vi "niRFUtil MT UTIL Generate Filter Coefficients.vi"(0 "System Filter Characteristic (none)":T1(ring), 1 "Modulation Type":T2(ring), 5 "Modulation Samples Per Symbol (16)":i32=16, 7 "Demodulation Samples Per Symbol (16)":i32=16, 9 "Filter Parameter":dbl=0.5 format="%.2f", 11 "error in (no error)":errorcluster, 12 "Filter Length (3)":i32=3) -> (4 "Pulse Shaping Filter Coefficients":T3 min=0 max=127 format="%.2f", 6 "Matched Filter Coefficients":T3 min=0 max=127 format="%.2f", 15 "error out":errorcluster)   [LabVIEW 2015, in "niRFUtil.lvlib"]
uses:
  niRFUtil.lvlib
  Includes/niRFUtil INC Real Array.ctl
  <vilib>/Analysis/2dsp.llb/1D Convolution (DBL).vi
  <vilib>/measure/masml.llb/ma_sml_Interpolation by Zero Insert (real input).vi
  <vilib>/Analysis/NI_AALPro.lvlib
  <vilib>/measure/NI_MAPro.lvlib
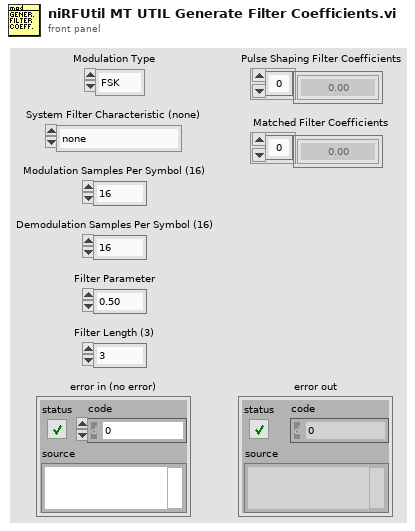
[diagram p1: front panel]
types:
  T1 = enum16{"none", "Raised Cosine", "Root Raised Cos", "Gaussian"}
  T2 = enum16{"FSK", "PSK", "QAM", "MSK", "PAM", "ASK", "CPM"}
  T3 = typedef "niRFUtil.lvlib/niRFUtil INC Real Array.ctl" = sgl[]
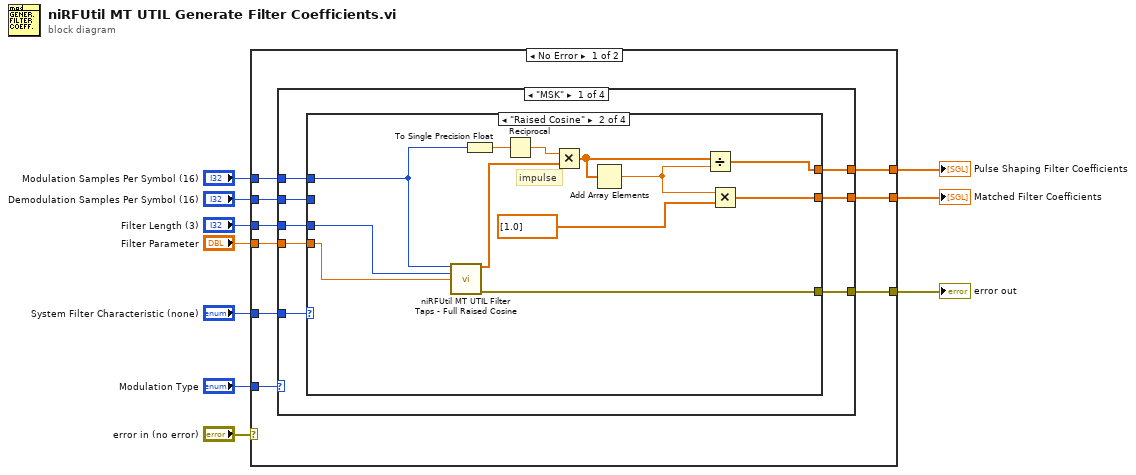
[diagram p0: block diagram]
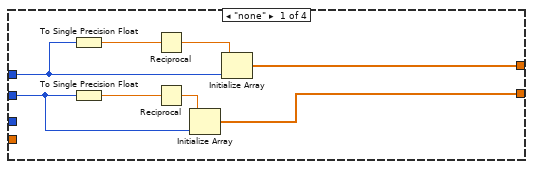
[diagram p2: hidden frame]
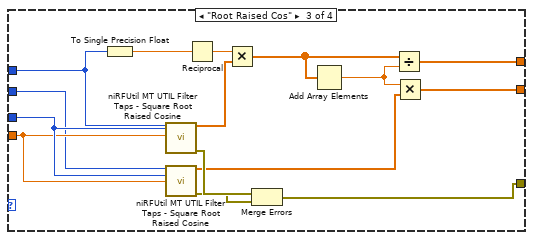
[diagram p3: hidden frame]
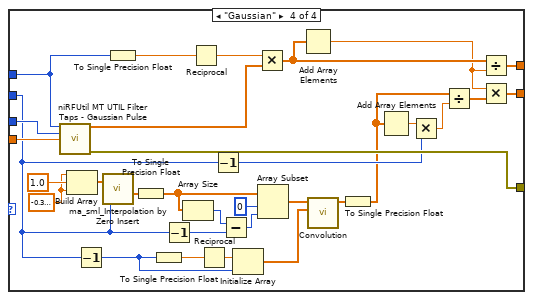
[diagram p4: hidden frame]
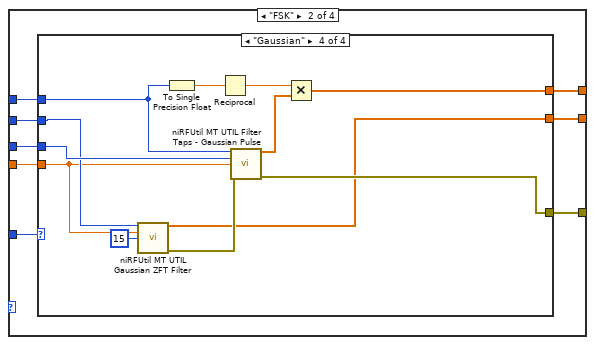
[diagram p5: hidden frame]
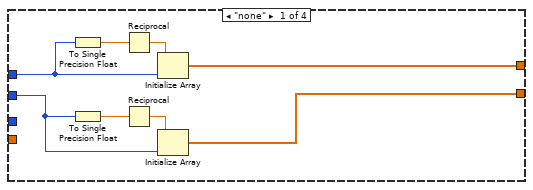
[diagram p6: hidden frame]
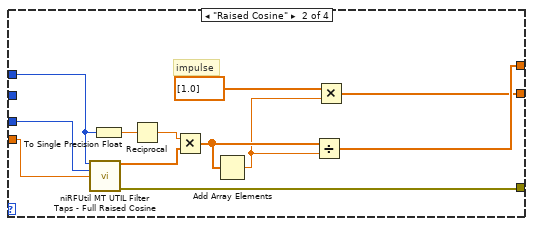
[diagram p7: hidden frame]
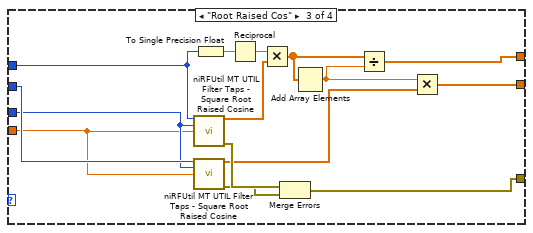
[diagram p8: hidden frame]
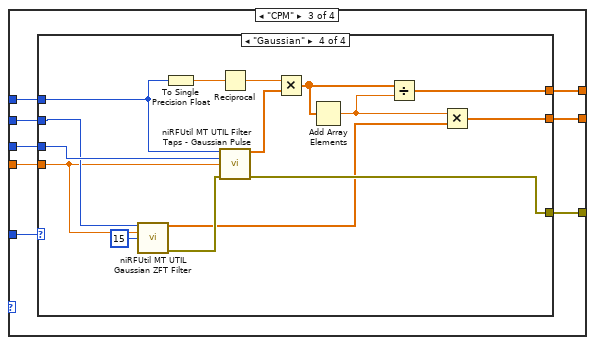
[diagram p9: hidden frame]
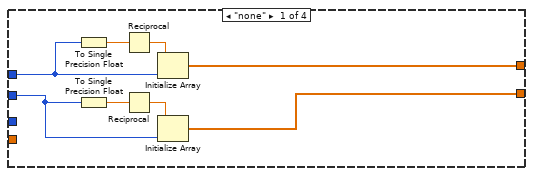
[diagram p10: hidden frame]
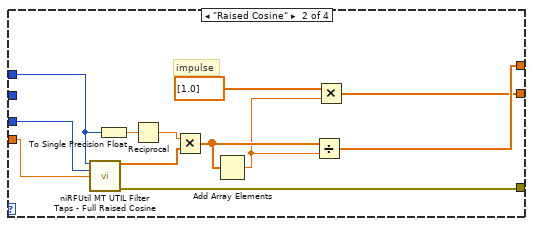
[diagram p11: hidden frame]
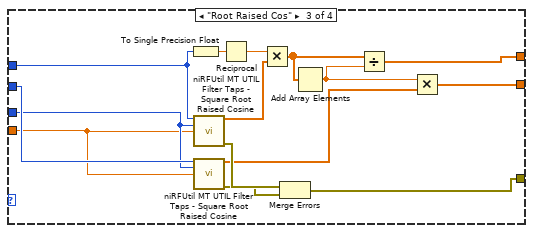
[diagram p12: hidden frame]
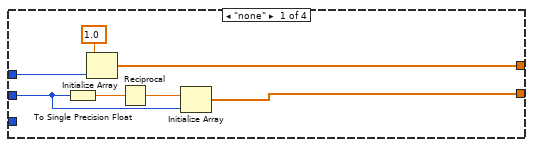
[diagram p14: hidden frame]
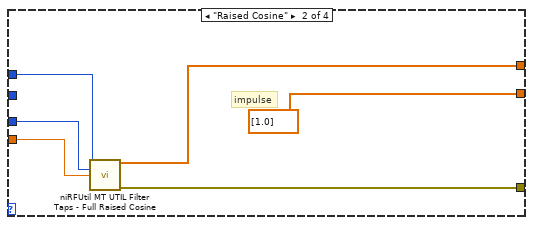
[diagram p15: hidden frame]
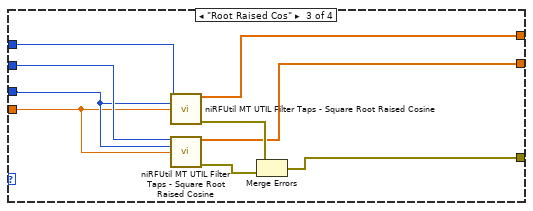
[diagram p16: hidden frame]
diagram:
  n1 = case shown="No Error" "error in (no error)" {
    selector: "error in (no error)" -> [_ w238]
    tunnel: [w19 _] -> w10
    tunnel: [w18 _] -> w9
    tunnel: "Demodulation Samples Per Symbol (16)" -> [w17 _]
    tunnel: "Modulation Type" -> [w16 _]
    tunnel: [w15 w238] -> w6
    tunnel: "Filter Parameter" -> [w14 _]
    tunnel: "Filter Length (3)" -> [w13 _]
    tunnel: "System Filter Characteristic (none)" -> [w12 _]
    tunnel: "Modulation Samples Per Symbol (16)" -> [w11 _]
    frame No Error {
      n2 = case shown="\"MSK\"" w16 {
        tunnel: w11 -> [w27 w102 w157 w215]
        tunnel: w12 -> [w26 w101 w156 w214]
        tunnel: w13 -> [w25 w100 w155 w213]
        tunnel: [w24 w99 w154 w212] -> w18
        tunnel: w14 -> [w23 w98 w153 w211]
        tunnel: [w22 w97 w152 w210] -> w15
        tunnel: w17 -> [w21 w96 w151 w209]
        tunnel: [w20 w95 w150 w208] -> w19
        frame "MSK" {
          n3 = case shown="\"Raised Cosine\"" w26 {
            tunnel: w27 -> [w30 w37 w49 w63]
            tunnel: w25 -> [_ w44 w59 w91]
            tunnel: w23 -> [_ w43 w58 w83]
            tunnel: [_ w45 w57 w93] -> w22
            tunnel: [w35 w41 w54 w71] -> w24
            tunnel: w21 -> [w29 _ w56 w76]
            tunnel: [w34 w38 w51 w70] -> w20
            frame "none" {
              n4 = To Single Precision Float(number=w30) -> (single precision float=w31:sgl)
              n5 = To Single Precision Float(number=w29) -> (single precision float=w28:sgl)
              n6 = Reciprocal(x=w31) -> (1/x=w33:sgl)
              n7 = Reciprocal(x=w28) -> (1/x=w32:sgl)
              n8 = Initialize Array(w32, w29) -> (w34:sgl[])
              n9 = Initialize Array(w33, w30) -> (w35:sgl[])
            }
            frame "Raised Cosine" {
              # "impulse"
              n10 = call "niRFUtil MT UTIL Filter Taps - Full Raised Cosine.vi"("Samples Per Symbol (16)"=w37, "Filter Length (3)"=w44, "Alpha (0.5)"=w43) -> ("Filter Coefficients"=w47:T3, "error out"=w45:errorcluster)  [unwired: 1 in, 10 out]
              n11 = To Single Precision Float(number=w37) -> (single precision float=w36:sgl)
              n12 = Reciprocal(x=w36) -> (1/x=w46:sgl)
              n13 = Multiply(x=w46, y=w47) -> (x*y=w42:T3)
              n14 = Add Array Elements(numeric array=w42) -> (sum=w40:sgl)
              n15 = Divide(x=w42, y=w40) -> (x/y=w41:T3)
              n16 = Multiply(x=w40, y=T3 [1.0]) -> (x*y=w38:T3)
            }
            frame "Root Raised Cos" {
              n17 = To Single Precision Float(number=w49) -> (single precision float=w48:sgl)
              n18 = call "niRFUtil MT UTIL Filter Taps - Square Root Raised Cosine.vi"("Samples Per Symbol (16)"=w49, "Filter Length (3)"=w59, "Alpha (0.5)"=w58) -> ("Filter Coefficients"=w55:T3, "error out"=w62:errorcluster)  [unwired: 1 in, 10 out]
              n19 = call "niRFUtil MT UTIL Filter Taps - Square Root Raised Cosine.vi"("Samples Per Symbol (16)"=w56, "Filter Length (3)"=w59, "Alpha (0.5)"=w58) -> ("Filter Coefficients"=w52:T3, "error out"=w61:errorcluster)  [unwired: 1 in, 10 out]
              n20 = Reciprocal(x=w48) -> (1/x=w60:sgl)
              n21 = Multiply(x=w60, y=w55) -> (x*y=w50:T3)
              n22 = Merge Errors(w62, w61) -> (w57:errorcluster)
              n23 = Add Array Elements(numeric array=w50) -> (sum=w53:sgl)
              n24 = Divide(x=w50, y=w53) -> (x/y=w54:T3)
              n25 = Multiply(x=w53, y=w52) -> (x*y=w51:T3)
            }
            frame "Gaussian" {
              w73 = sgl -0.3
              n26 = call "niRFUtil MT UTIL Filter Taps - Gaussian Pulse.vi"("Samples Per Symbol (16)"=w63, "Filter Length (3)"=w91, "Alpha (0.5)"=w83) -> ("Filter Coefficients"=w94:T3, "error out"=w93:errorcluster)  [unwired: 1 in, 10 out]
              n27 = Build Array(w73, sgl 1.0, w73) -> (w82:sgl[])
              n28 = Decrement(x=w76) -> (x-1=w66:i32)
              n29 = call-poly <vilib>:"ma_sml_Interpolation by Zero Insert.vi"("L"=w76, "x"=w82) -> ("y"=w87:dbl[])
              n30 = To Single Precision Float(number=w63) -> (single precision float=w64:sgl)
              n31 = To Single Precision Float(number=w87) -> (single precision float=w68:sgl[])
              n32 = To Single Precision Float(number=w66) -> (single precision float=w67:sgl)
              n33 = Decrement(x=w76) -> (x-1=w84:i32)
              n34 = Array Size(array=w68) -> (size(s)=w86:i32)
              n35 = Reciprocal(x=w64) -> (1/x=w92:sgl)
              n36 = Reciprocal(x=w67) -> (1/x=w90:sgl)
              n37 = Decrement(x=w76) -> (x-1=w77:i32)
              n38 = Subtract(x=w86, y=w84) -> (x-y=w85:i32)
              n39 = Initialize Array(w90, w66) -> (w75:sgl[])
              n40 = Multiply(x=w92, y=w94) -> (x*y=w72:T3)
              n41 = Array Subset(array=w68, index=0, length=w85) -> (w81:sgl[])
              n42 = Add Array Elements(numeric array=w72) -> (sum=w69:sgl)
              n43 = call-poly <vilib>:"Convolution.vi"("Y"=w75, "X"=w81) -> ("X * Y"=w80:dbl[])  [unwired: 1 in, 8 out]
              n44 = To Single Precision Float(number=w80) -> (single precision float=w65:sgl[])
              n45 = Add Array Elements(numeric array=w65) -> (sum=w79:sgl)
              n46 = Multiply(x=w79, y=w77) -> (x*y=w78:sgl)
              n47 = Divide(x=w65, y=w78) -> (x/y=w74:sgl[])
              n48 = Divide(x=w72, y=w69) -> (x/y=w71:T3)
              n49 = Multiply(x=w69, y=w74) -> (x*y=w70:sgl[])
            }
          }
        }
        frame "FSK" {
          n50 = case shown="\"Gaussian\"" w101 {
            tunnel: w102 -> [w106 w112 w124 w139]
            tunnel: w100 -> [_ w122 w134 w146]
            tunnel: w98 -> [_ w121 w133 w141]
            tunnel: [_ w118 w131 w148] -> w97
            tunnel: [w110 w116 w129 w145] -> w99
            tunnel: w96 -> [w104 _ w135 w144]
            tunnel: [w109 w113 w126 w142] -> w95
            frame "none" {
              n51 = To Single Precision Float(number=w106) -> (single precision float=w105:sgl)
              n52 = To Single Precision Float(number=w104) -> (single precision float=w103:sgl)
              n53 = Reciprocal(x=w105) -> (1/x=w108:sgl)
              n54 = Reciprocal(x=w103) -> (1/x=w107:sgl)
              n55 = Initialize Array(w108, w106) -> (w110:sgl[])
              n56 = Initialize Array(w107, w104) -> (w109:sgl[])
            }
            frame "Raised Cosine" {
              # "impulse"
              n57 = call "niRFUtil MT UTIL Filter Taps - Full Raised Cosine.vi"("Samples Per Symbol (16)"=w112, "Filter Length (3)"=w122, "Alpha (0.5)"=w121) -> ("Filter Coefficients"=w120:T3, "error out"=w118:errorcluster)  [unwired: 1 in, 10 out]
              n58 = To Single Precision Float(number=w112) -> (single precision float=w111:sgl)
              n59 = Reciprocal(x=w111) -> (1/x=w119:sgl)
              n60 = Multiply(x=w119, y=w120) -> (x*y=w117:T3)
              n61 = Add Array Elements(numeric array=w117) -> (sum=w115:sgl)
              n62 = Divide(x=w117, y=w115) -> (x/y=w116:T3)
              n63 = Multiply(x=T3 [1.0], y=w115) -> (x*y=w113:T3)
            }
            frame "Root Raised Cos" {
              n64 = call "niRFUtil MT UTIL Filter Taps - Square Root Raised Cosine.vi"("Samples Per Symbol (16)"=w124, "Filter Length (3)"=w134, "Alpha (0.5)"=w133) -> ("Filter Coefficients"=w130:T3, "error out"=w137:errorcluster)  [unwired: 1 in, 10 out]
              n65 = call "niRFUtil MT UTIL Filter Taps - Square Root Raised Cosine.vi"("Samples Per Symbol (16)"=w135, "Filter Length (3)"=w134, "Alpha (0.5)"=w133) -> ("Filter Coefficients"=w127:T3, "error out"=w136:errorcluster)  [unwired: 1 in, 10 out]
              n66 = To Single Precision Float(number=w124) -> (single precision float=w123:sgl)
              n67 = Reciprocal(x=w123) -> (1/x=w132:sgl)
              n68 = Multiply(x=w132, y=w130) -> (x*y=w125:T3)
              n69 = Merge Errors(w137, w136) -> (w131:errorcluster)
              n70 = Add Array Elements(numeric array=w125) -> (sum=w128:sgl)
              n71 = Divide(x=w125, y=w128) -> (x/y=w129:T3)
              n72 = Multiply(x=w128, y=w127) -> (x*y=w126:T3)
            }
            frame "Gaussian" {
              n73 = call "niRFUtil MT UTIL Gaussian ZFT Filter.vi"("Samples Per Symbol (16)"=w144, "Filter Parameter"=w141, "Filter Length (3)"=15) -> ("Demod Filter Taps"=w142:T3, "error out"=w143:errorcluster)  [unwired: 1 in, 10 out]
              n74 = To Single Precision Float(number=w139) -> (single precision float=w138:sgl)
              n75 = Reciprocal(x=w138) -> (1/x=w147:sgl)
              n76 = call "niRFUtil MT UTIL Filter Taps - Gaussian Pulse.vi"("Samples Per Symbol (16)"=w139, "Filter Length (3)"=w146, "Alpha (0.5)"=w141, "error in (no error)"=w143) -> ("Filter Coefficients"=w149:T3, "error out"=w148:errorcluster)  [unwired: 10 out]
              n77 = Multiply(x=w147, y=w149) -> (x*y=w145:T3)
            }
          }
        }
        frame "CPM" {
          n78 = case shown="\"Gaussian\"" w156 {
            tunnel: w157 -> [w161 w167 w179 w194]
            tunnel: w155 -> [_ w177 w189 w204]
            tunnel: w153 -> [_ w176 w188 w201]
            tunnel: [_ w173 w186 w206] -> w152
            tunnel: [w165 w171 w184 w197] -> w154
            tunnel: w151 -> [w159 _ w190 w203]
            tunnel: [w164 w168 w181 w195] -> w150
            frame "none" {
              n79 = To Single Precision Float(number=w161) -> (single precision float=w160:sgl)
              n80 = To Single Precision Float(number=w159) -> (single precision float=w158:sgl)
              n81 = Reciprocal(x=w160) -> (1/x=w163:sgl)
              n82 = Reciprocal(x=w158) -> (1/x=w162:sgl)
              n83 = Initialize Array(w163, w161) -> (w165:sgl[])
              n84 = Initialize Array(w162, w159) -> (w164:sgl[])
            }
            frame "Raised Cosine" {
              # "impulse"
              n85 = call "niRFUtil MT UTIL Filter Taps - Full Raised Cosine.vi"("Samples Per Symbol (16)"=w167, "Filter Length (3)"=w177, "Alpha (0.5)"=w176) -> ("Filter Coefficients"=w175:T3, "error out"=w173:errorcluster)  [unwired: 1 in, 10 out]
              n86 = To Single Precision Float(number=w167) -> (single precision float=w166:sgl)
              n87 = Reciprocal(x=w166) -> (1/x=w174:sgl)
              n88 = Multiply(x=w174, y=w175) -> (x*y=w172:T3)
              n89 = Add Array Elements(numeric array=w172) -> (sum=w170:sgl)
              n90 = Divide(x=w172, y=w170) -> (x/y=w171:T3)
              n91 = Multiply(x=T3 [1.0], y=w170) -> (x*y=w168:T3)
            }
            frame "Root Raised Cos" {
              n92 = To Single Precision Float(number=w179) -> (single precision float=w178:sgl)
              n93 = call "niRFUtil MT UTIL Filter Taps - Square Root Raised Cosine.vi"("Samples Per Symbol (16)"=w179, "Filter Length (3)"=w189, "Alpha (0.5)"=w188) -> ("Filter Coefficients"=w185:T3, "error out"=w192:errorcluster)  [unwired: 1 in, 10 out]
              n94 = call "niRFUtil MT UTIL Filter Taps - Square Root Raised Cosine.vi"("Samples Per Symbol (16)"=w190, "Filter Length (3)"=w189, "Alpha (0.5)"=w188) -> ("Filter Coefficients"=w182:T3, "error out"=w191:errorcluster)  [unwired: 1 in, 10 out]
              n95 = Reciprocal(x=w178) -> (1/x=w187:sgl)
              n96 = Multiply(x=w187, y=w185) -> (x*y=w180:T3)
              n97 = Merge Errors(w192, w191) -> (w186:errorcluster)
              n98 = Add Array Elements(numeric array=w180) -> (sum=w183:sgl)
              n99 = Divide(x=w180, y=w183) -> (x/y=w184:T3)
              n100 = Multiply(x=w183, y=w182) -> (x*y=w181:T3)
            }
            frame "Gaussian" {
              n101 = call "niRFUtil MT UTIL Gaussian ZFT Filter.vi"("Samples Per Symbol (16)"=w203, "Filter Parameter"=w201, "Filter Length (3)"=15) -> ("Demod Filter Taps"=w196:T3, "error out"=w202:errorcluster)  [unwired: 1 in, 10 out]
              n102 = To Single Precision Float(number=w194) -> (single precision float=w193:sgl)
              n103 = Reciprocal(x=w193) -> (1/x=w205:sgl)
              n104 = call "niRFUtil MT UTIL Filter Taps - Gaussian Pulse.vi"("Samples Per Symbol (16)"=w194, "Filter Length (3)"=w204, "Alpha (0.5)"=w201, "error in (no error)"=w202) -> ("Filter Coefficients"=w207:T3, "error out"=w206:errorcluster)  [unwired: 10 out]
              n105 = Multiply(x=w205, y=w207) -> (x*y=w198:T3)
              n106 = Add Array Elements(numeric array=w198) -> (sum=w199:sgl)
              n107 = Divide(x=w198, y=w199) -> (x/y=w197:T3)
              n108 = Multiply(x=w199, y=w196) -> (x*y=w195:T3)
            }
          }
        }
        frame "PSK", "QAM", "PAM", "ASK", Default {
          n109 = case shown="\"Gaussian\"" w214 {
            tunnel: w215 -> [w221 w226 w236 _]
            tunnel: w213 -> [_ w225 w234 _]
            tunnel: w211 -> [_ w224 w233 _]
            tunnel: [_ w228 w229 _] -> w210
            tunnel: [w220 w227 w237 _] -> w212
            tunnel: w209 -> [w217 _ w235 _]
            tunnel: [w218 T3 [1.0] w231 _] -> w208
            frame "none" {
              n110 = To Single Precision Float(number=w217) -> (single precision float=w216:sgl)
              n111 = Initialize Array(sgl 1.0 ("Element Data"), w221) -> (w220:sgl[])
              n112 = Reciprocal(x=w216) -> (1/x=w219:sgl)
              n113 = Initialize Array(w219, w217) -> (w218:sgl[])
            }
            frame "Raised Cosine" {
              # "impulse"
              n114 = call "niRFUtil MT UTIL Filter Taps - Full Raised Cosine.vi"("Samples Per Symbol (16)"=w226, "Filter Length (3)"=w225, "Alpha (0.5)"=w224) -> ("Filter Coefficients"=w227:T3, "error out"=w228:errorcluster)  [unwired: 1 in, 10 out]
            }
            frame "Root Raised Cos" {
              n115 = call "niRFUtil MT UTIL Filter Taps - Square Root Raised Cosine.vi"("Samples Per Symbol (16)"=w236, "Filter Length (3)"=w234, "Alpha (0.5)"=w233) -> ("Filter Coefficients"=w237:T3, "error out"=w232:errorcluster)  [unwired: 1 in, 10 out]
              n116 = call "niRFUtil MT UTIL Filter Taps - Square Root Raised Cosine.vi"("Samples Per Symbol (16)"=w235, "Filter Length (3)"=w234, "Alpha (0.5)"=w233) -> ("Filter Coefficients"=w231:T3, "error out"=w230:errorcluster)  [unwired: 1 in, 10 out]
              n117 = Merge Errors(w232, w230) -> (w229:errorcluster)
            }
            frame "Gaussian" {
              # "not allowed"
            }
          }
        }
      }
    }
    frame Error {
    }
  }
  "Matched Filter Coefficients" <- w10
  "Pulse Shaping Filter Coefficients" <- w9
  "error out" <- w6
